vi "WinCI Get Project Name.vi"(2 "config data in":string) -> (7 "project name":string)   [LabVIEW 2020, in "NI_SCC_WinCI.lvlib"]
uses:
  <vilib>/SourceControl/Providers/WinCI/NI_SCC_WinCI.lvlib
  <vilib>/SourceControl/support/SCCSup ConfigData Conv.ctl
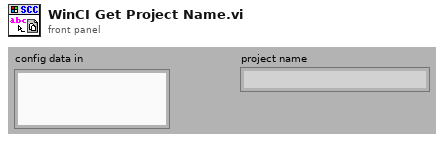
[diagram p1: front panel]
types:
  T1 = typedef "SCCSup ConfigData Conv.ctl" = enum16{"from config data", "to config data"}
  T2 = typedef "NI_SCC_WinCI.lvlib/WinCI SCC Project Details.ctl" = cluster{"user name":string, "project name":string, "local path":string, "database name":string}
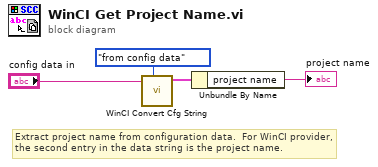
[diagram p0: block diagram]
diagram:
  # "Extract project name from configuration data.  For WinCI provider, the second entry in the data string is the project name."
  n1 = call <vilib>:"WinCI Convert Cfg String.vi"("conversion action"=SCCSup_ConfigData_Conv."from config data", "config data in"="config data in") -> ("project details out"=w2:T2)  [unwired: 1 in, 8 out]
  n2 = Unbundle By Name(w2) -> ("project name"=→"project name":string)
